vi "Channel Parameters List.vi"(8 "error in (no error)":errorcluster, 10 "Channel (0)":u8, 11 "BoardHandle":T1) -> (0 "error out":errorcluster, 1 "Status bits":string[](array[string]), 2 "Parameters list":string[](array[string]), 3 "BoardHandle out":T1)   [LabVIEW 2020, in "CAEN PSM.lvlib"]
doc: "This function returns the list of channel parameters supported by the device."
uses:
  CAEN PSM.lvlib
  Private/BoardHandle.ctl
  Private/DeviceFamily.ctl
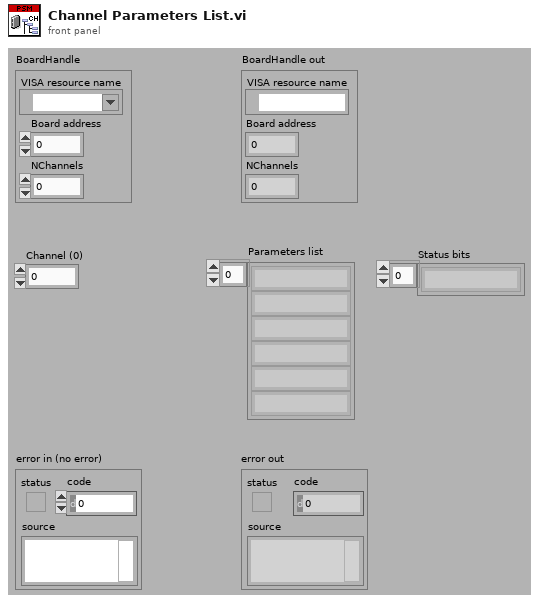
[diagram p1: front panel]
types:
  T1 = typedef "CAEN PSM.lvlib/BoardHandle.ctl" = cluster{"VISA resource name":refnum<visa-resource-name>, "Board address":i8, "NChannels":u8}
  T2 = typedef "CAEN PSM.lvlib/DeviceFamily.ctl" = enum8{"NIM / DESKTOP HV", "DT55XXE HV", "SMART HV"}
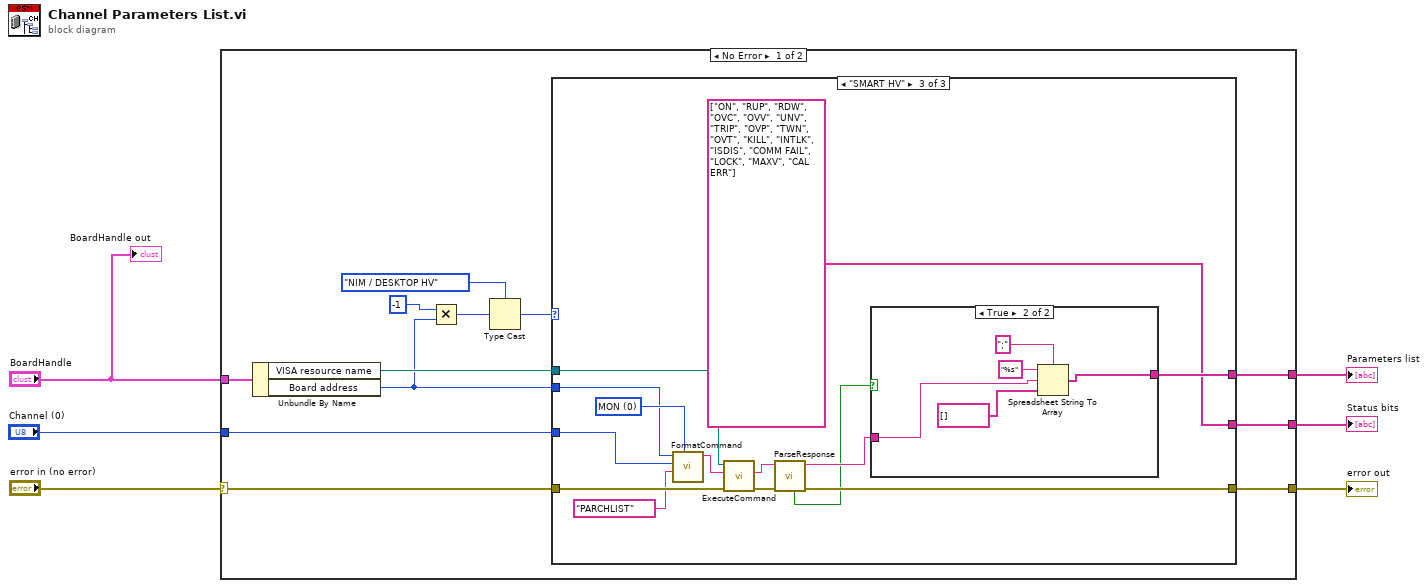
[diagram p0: block diagram]
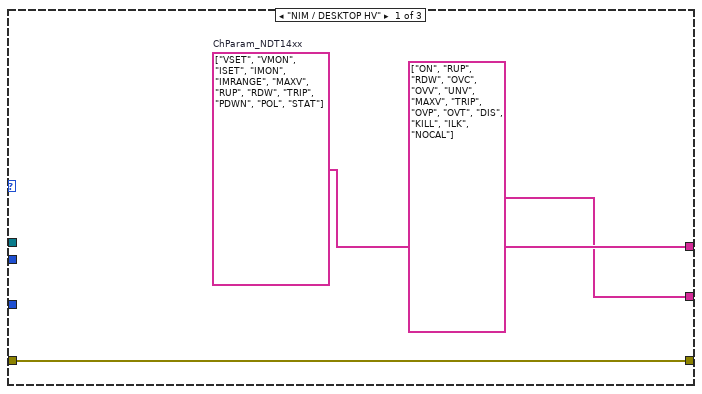
[diagram p2: hidden frame]
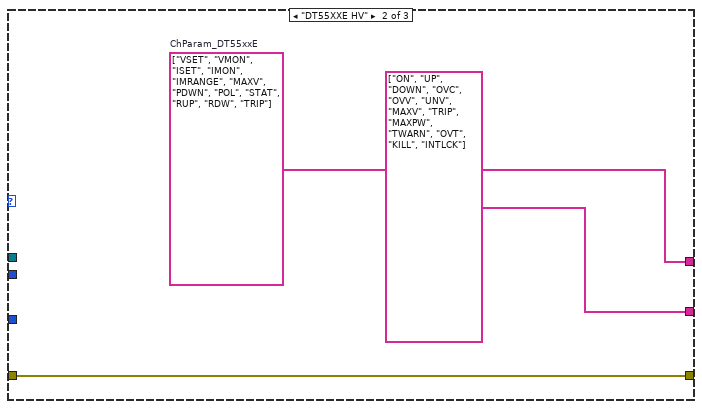
[diagram p3: hidden frame]
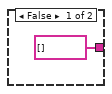
[diagram p4: hidden frame]
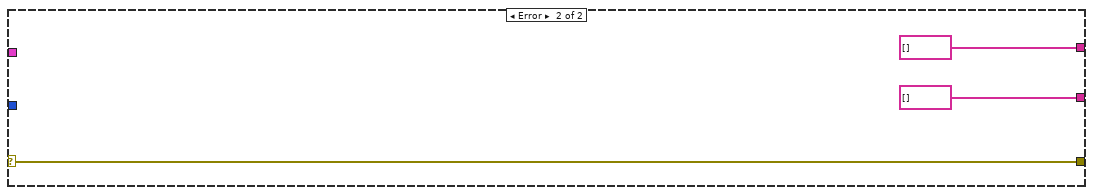
[diagram p5: hidden frame]
diagram:
  n1 = case shown="No Error" "error in (no error)" {
    selector: "error in (no error)" -> [w17 w47]
    tunnel: [w14 w47] -> w5
    tunnel: "BoardHandle" -> [w18 _]
    tunnel: "Channel (0)" -> [w15 _]
    tunnel: [w13 string[] [] ("array type (2D Dbl)")] -> w2
    tunnel: [w10 string[] []] -> w1
    frame No Error {
      n2 = Unbundle By Name(w18) -> ("VISA resource name"=w16:refnum<visa-resource-name>, "Board address"=w8:i8)
      n3 = Multiply(x=i8 -1, y=w8) -> (x*y=w9:i8)
      n4 = Type Cast(type=DeviceFamily."NIM / DESKTOP HV" ("Device Family"), x=w9) -> (*(type *) &x=w11:T2)
      n5 = case shown="\"SMART HV\"" w11 {
        tunnel: w17 -> [w21 w24 w34]
        tunnel: w16 -> [_ _ w33]
        tunnel: w8 -> [_ _ w32]
        tunnel: w15 -> [_ _ w31]
        tunnel: [w21 w24 w29] -> w14
        tunnel: [w20 w23 w26] -> w13
        tunnel: [string[] ["ON", "RUP", "RDW", "OVC", "OVV", "UNV", "MAXV", "TRIP", "OVP", "OVT", "DIS", "KILL", "ILK", "NOCAL"] string[] ["ON", "UP", "DOWN", "OVC", "OVV", "UNV", "MAXV", "TRIP", "MAXPW", "TWARN", "OVT", "KILL", "INTLCK"] string[] ["ON", "RUP", "RDW", "OVC", "OVV", "UNV", "TRIP", "OVP", "TWN", "OVT", "KILL", "INTLK", "ISDIS", "COMM FAIL", "LOCK", "MAXV", "CAL ERR"]] -> w10
        frame "NIM / DESKTOP HV" {
          w20 = string[] ["VSET", "VMON", "ISET", "IMON", "IMRANGE", "MAXV", "RUP", "RDW", "TRIP", "PDWN", "POL", "STAT"]  # ChParam_NDT14xx
        }
        frame "DT55XXE HV" {
          w23 = string[] ["VSET", "VMON", "ISET", "IMON", "IMRANGE", "MAXV", "PDWN", "POL", "STAT", "RUP", "RDW", "TRIP"]  # ChParam_DT55xxE
        }
        frame "SMART HV" {
          w38 = u8 0 items=["MON", "SET"] ("CMD")
          n6 = call "FormatCommand.vi"("CMD (MON)"=w38, "PAR"="PARCHLIST", "CH"=w31, "BD (0)"=w32) -> ("cmd"=w37:string)  [unwired: 7 in]
          n7 = call "ExecuteCommand.vi"("error in (no error)"=w34, "Command"=w37, "VISA resource name"=w33) -> ("error out"=w36:errorcluster, "Response"=w35:string)  [unwired: 6 in, 1 out]
          n8 = call "ParseResponse.vi"("error in (no error)"=w36, "Response"=w35) -> ("error out"=w29:errorcluster, "val"=w28:string, "OK"=w27:bool)  [unwired: 6 in, 1 out]
          n9 = case shown="True" w27 {
            tunnel: w28 -> [_ w42]
            tunnel: [string[] [] ("array type (2D Dbl)") w40] -> w26
            frame False {
            }
            frame True {
              n10 = Spreadsheet String To Array(delimiter (Tab)=";", format string="%s", spreadsheet string=w42, array type (2D Dbl)=string[] []) -> (array=w40:string[])
            }
          }
        }
      }
    }
    frame Error {
    }
  }
  "error out" <- w5
  "Parameters list" <- w2
  "Status bits" <- w1
  "BoardHandle out" <- "BoardHandle"
